vi "远程本地T.vi"() -> ()   [LabVIEW 2015]
panel:
  in  "登陆次数":dbl
  out "远程本地":T1
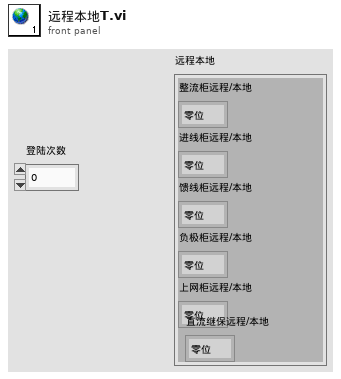
[diagram p1: front panel]
types:
  T1 = cluster{"整流柜远程/本地":enum16{"零位", "本地", "远方"}, "进线柜远程/本地":enum16{"零位", "本地", "远方"}, "馈线柜远程/本地":enum16{"零位", "本地", "远方"}, "负极柜远程/本地":enum16{"零位", "本地", "远方"}, "上网柜远程/本地":enum16{"零位", "本地", "远方"}, "直流继保远程/本地":enum16{"零位", "本地", "远方"}}
diagram:
